vi "Pre Launch Init.vi"(11 "Async Methods Actor in":refnum<class "Async Methods Actor.lvclass">) -> (0 "error out":errorcluster, 3 "Async Methods Actor out":refnum<class "Async Methods Actor.lvclass">)   [LabVIEW 2021, in "Async Methods Actor.lvlib" / "Async Methods Actor.lvclass"]
doc: "(<B>Filename</B>: Actor Framework.lvlib:Actor.lvclass:Pre Launch Init.vi)\n\nDefines behavior that occurs after the Launch Nested Actor method is invoked but before the actor's Actor Core method begins running.\n\nBy default, this method does nothing. A descendant class may override it to define behavior."
uses:
  Async Methods Actor.lvclass
  Async Methods Running.ctl
  Async Message Execution Status Map.ctl
  Async Message Execution Status.ctl
  VI Refnums Map.ctl
  VI Refnums Map Value.ctl
  Async Call Method.ctl
  Async Methods Actor.lvclass/Async Methods Actor.ctl
  78a32560-03ad-477a-8f36-c16de347af0f.vi
  51009067-ad9f-4da9-820d-fc8521565866.vi
  <vilib>/ActorFramework/Actor/Actor.lvclass
  Async Methods Actor Messages/Async Message/Async Message.lvclass
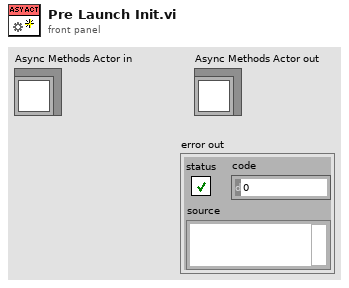
[diagram p1: front panel]
types:
  T1 = typedef "Async Methods Actor.lvlib/Async Methods Actor.lvclass/Async Methods Running.ctl" = cluster{"Async Messages":string[], "C&C Running":u32[], "C&F Launched":u32[]}
  T2 = typedef "Async Methods Actor.lvlib/Async Methods Actor.lvclass/Async Message Execution Status Map.ctl" = map{string, T3}
  T3 = typedef "Async Methods Actor.lvlib/Async Methods Actor.lvclass/Async Message Execution Status.ctl" = cluster{"C&C Clones Running":u32, "C&F Clones Launched":u32}
  T4 = typedef "Async Methods Actor.lvlib/Async Methods Actor.lvclass/VI Refnums Map.ctl" = map{refnum<vi>, T5}
  T5 = typedef "Async Methods Actor.lvlib/Async Methods Actor.lvclass/VI Refnums Map Value.ctl" = cluster{"Async Call Method":T6, "Message Path":path}
  T6 = typedef "Async Methods Actor.lvlib/Async Methods Actor.lvclass/Async Call Method.ctl" = enum16{"Call and Collect", "Call and Forget"}
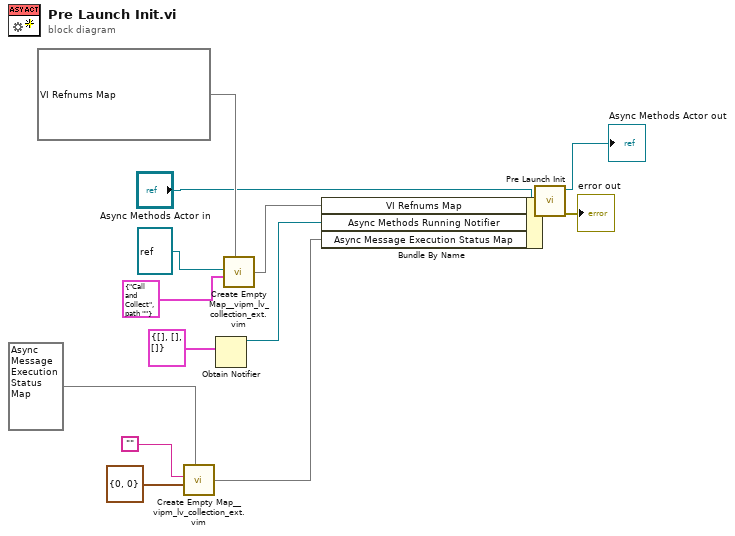
[diagram p0: block diagram]
diagram:
  n1 = call "Create Empty Map__vipm_lv_collection_ext.vim"("value type"=T3 {"C&C Clones Running"=0, "C&F Clones Launched"=0} ("Async Message Execution Status"), "map type (optional)"=T2 {} ("Async Message Execution Status Map"), "key type"="") -> ("empty map"=w7:T2)  [unwired: 7 in]
  n2 = Obtain Notifier(notification data type=T1 {"Async Messages"=[], "C&C Running"=[], "C&F Launched"=[]} ("Async Methods Running")) -> (notifier out=w4:refnum<notifier>)  [unwired: 3 in, 2 out]
  n3 = call "Create Empty Map__vipm_lv_collection_ext.vim"("value type"=T5 {"Async Call Method"=enum."Call and Collect", "Message Path"=path ""} ("VI Refnums Map Value"), "map type (optional)"=T4 {} ("VI Refnums Map"), "key type"=refnum<vi> refnum ("type specifier VI Refnum (for type only)")) -> ("empty map"=w10:T4)  [unwired: 7 in]
  n4 = Bundle By Name(cluster="Async Methods Actor in", "VI Refnums Map"=w10, "Async Methods Running Notifier"=w4, "Async Message Execution Status Map"=w7) -> (w13:refnum<class "Async Methods Actor.lvclass">)
  n5 = call-parent "Pre Launch Init.vi"("Actor in"=w13) -> ("error out"=→"error out":errorcluster, "Actor out"=→"Async Methods Actor out":refnum<class "Async Methods Actor.lvclass">)  [unwired: 9 in]
